vi "ReadSMUs.vi"(8 "Error In":errorcluster, 10 "Measure Configurations":T1[](array[typedef]) {"Count" min=1 step=1}, 11 "Keithley 2602 In":refnum<visa-resource-name>) -> (0 "Error Out":errorcluster, 3 "Keithley 2602 Out":refnum<visa-resource-name>)   [LabVIEW 2013]
uses:
  MeasureConfiguration.ctl
  driver/Public/Controls/SMU.ctl
  driver/Keithley-2602.lvlib
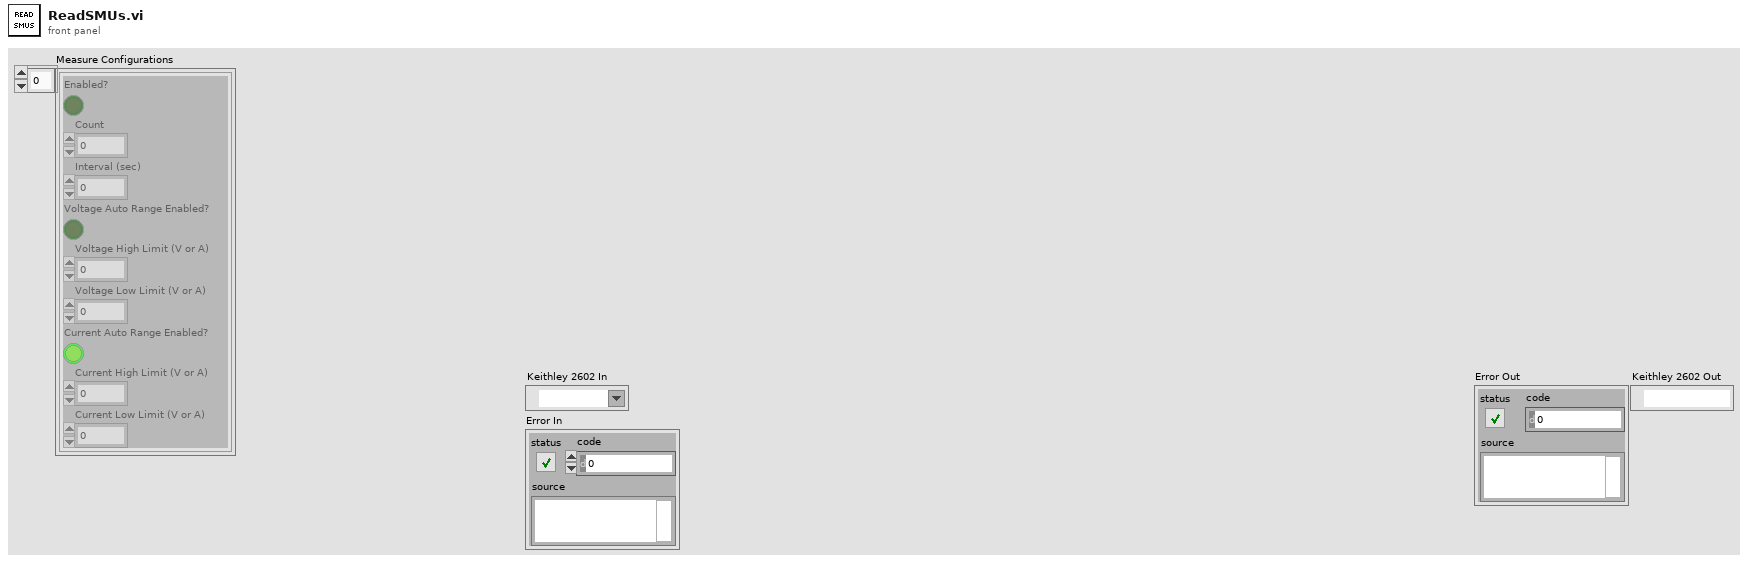
[diagram p1: front panel]
types:
  T1 = typedef "MeasureConfiguration.ctl" = cluster{"Enabled?":bool, "Count":u8, "Interval (sec)":dbl, "Voltage Auto Range Enabled?":bool, "Voltage High Limit (V or A)":dbl, "Voltage Low Limit (V or A)":dbl, "Current Auto Range Enabled?":bool, "Current High Limit (V or A)":dbl, "Current Low Limit (V or A)":dbl}
  T2 = typedef "Keithley-2602.lvlib/SMU.ctl" = enum16{"A", "B"}
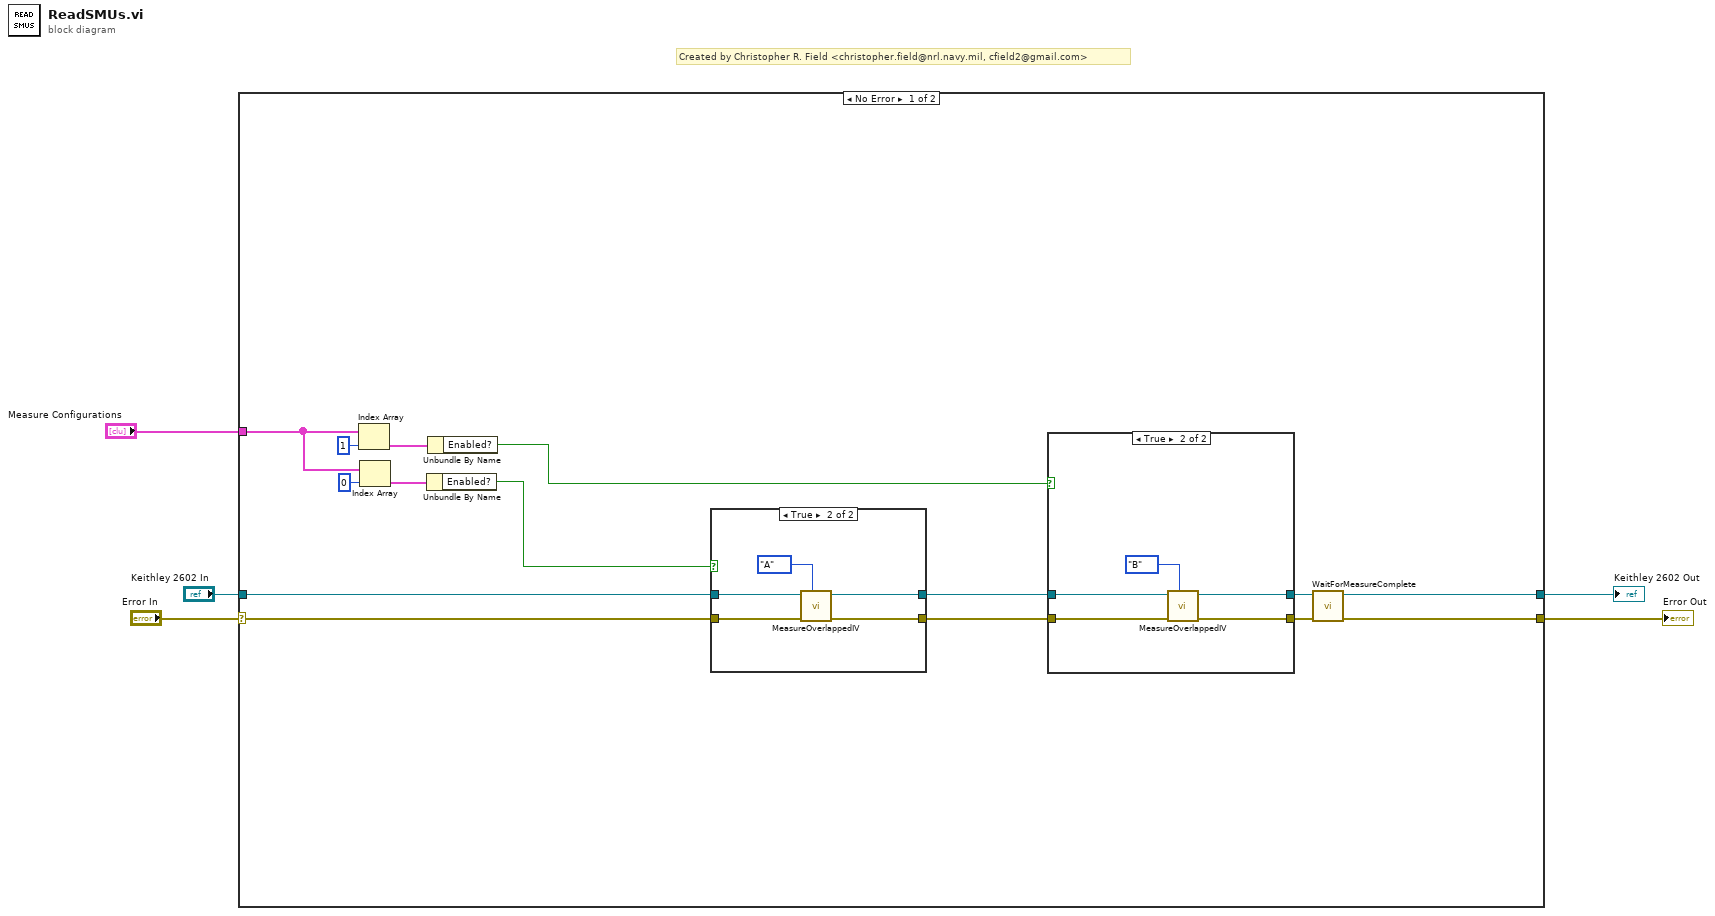
[diagram p0: block diagram]
diagram:
  # "Created by Christopher R. Field <christopher.field@nrl.navy.mil, cfield2@gmail.com>"
  n1 = case shown="No Error" "Error In" {
    selector: "Error In" -> [w17 w35]
    tunnel: "Keithley 2602 In" -> [w18 w36]
    tunnel: [w14 w35] -> w3
    tunnel: [w15 w36] -> w2
    tunnel: "Measure Configurations" -> [w10 _]
    frame No Error {
      n2 = Index Array(array=w10, index=1) -> (element=w9:T1)
      n3 = Index Array(array=w10, index=0) -> (element=w7:T1)
      n4 = Unbundle By Name(w7) -> ("Enabled?"=w6:bool)
      n5 = Unbundle By Name(w9) -> ("Enabled?"=w8:bool)
      n6 = case shown="True" w6 {
        tunnel: w18 -> [w22 w27]
        tunnel: w17 -> [w21 w26]
        tunnel: [w22 w25] -> w20
        tunnel: [w21 w24] -> w19
        frame False {
        }
        frame True {
          n7 = call "MeasureOverlappedIV.vi"("SMU"=SMU."A", "Error In"=w26, "Keithley 2602 In"=w27) -> ("Error Out"=w24:errorcluster, "Keithley 2602 Out"=w25:refnum<visa-resource-name>)  [unwired: 7 in]
        }
      }
      n8 = case shown="True" w8 {
        tunnel: w20 -> [w29 w34]
        tunnel: w19 -> [w28 w33]
        tunnel: [w29 w31] -> w16
        tunnel: [w28 w32] -> w13
        frame False {
        }
        frame True {
          n9 = call "MeasureOverlappedIV.vi"("SMU"=SMU."B", "Error In"=w33, "Keithley 2602 In"=w34) -> ("Error Out"=w32:errorcluster, "Keithley 2602 Out"=w31:refnum<visa-resource-name>)  [unwired: 7 in]
        }
      }
      n10 = call "WaitForMeasureComplete.vi"("Error In"=w13, "Keithley 2602 In"=w16) -> ("Error Out"=w14:errorcluster, "Keithley 2602 Out"=w15:refnum<visa-resource-name>)  [unwired: 8 in]
    }
    frame Error {
    }
  }
  "Error Out" <- w3
  "Keithley 2602 Out" <- w2
